vi "Close Text Log File.vi"(8 "error in (no error)":errorcluster, 11 "Text Log File in":refnum<class "Text Log File.lvclass">) -> (0 "error out":errorcluster, 3 "File Path":path)   [LabVIEW 2012, in "Waveform Data Logger Engine.lvlib" / "Text Log File.lvclass"]
uses:
  Text Log File.lvclass
  Text Log File.lvclass/Text Log File.ctl
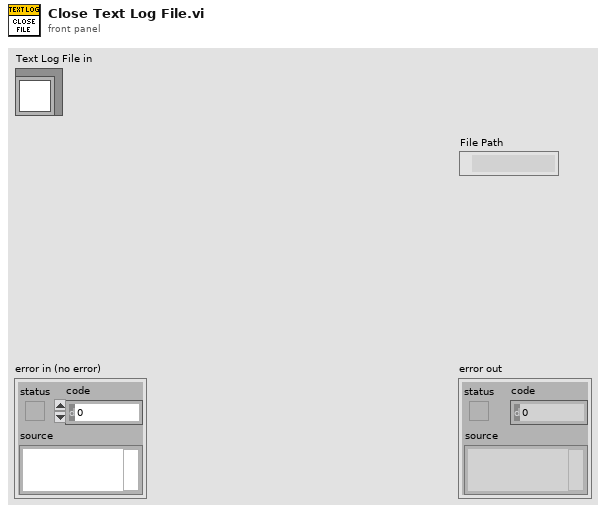
[diagram p1: front panel]
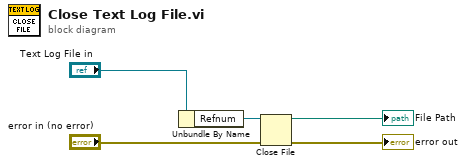
[diagram p0: block diagram]
diagram:
  n1 = Unbundle By Name("Text Log File in") -> ("Refnum"=w5:refnum<file>)
  n2 = Close File(refnum=w5, error in="error in (no error)") -> (path=→"File Path":path, error out=→"error out":errorcluster)
